vi "RGB to Colour.vi"(8 "error in (no error)":errorcluster, 9 "Blue":u8, 10 "Green":u8, 11 "Red":u8) -> (0 "error out":errorcluster, 3 "Color":u32(colorbox))   [LabVIEW 2018]
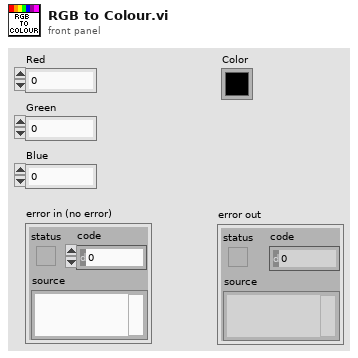
[diagram p1: front panel]
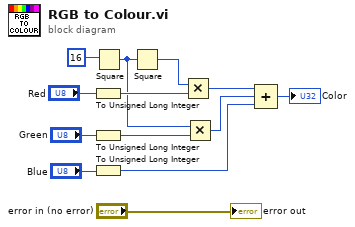
[diagram p0: block diagram]
diagram:
  n1 = To Unsigned Long Integer(number="Red") -> (unsigned 32bit integer=w9:u32)
  n2 = To Unsigned Long Integer(number="Green") -> (unsigned 32bit integer=w5:u32)
  n3 = To Unsigned Long Integer(number="Blue") -> (unsigned 32bit integer=w2:u32)
  n4 = Square(x=u32 16) -> (x^2=w3:u32)
  n5 = Square(x=w3) -> (x^2=w8:u32)
  n6 = Multiply(x=w8, y=w9) -> (x*y=w6:u32)
  n7 = Multiply(x=w3, y=w5) -> (x*y=w4:u32)
  n8 = Compound Arithmetic op=ADD(w6, w4, w2) -> (→"Color":u32)
  "error out" <- "error in (no error)"
